vi "RFmx Update Sweep - TOI.vi"(8 "error in (no error)":errorcluster, 10 "Current Settings":T1={"Pin per Tone (dBm)"=0.0, "Equivalent Pin Power (dBm)"=0.0, "Frequency (Hz)"=0.0, "Tone Spacing (Hz)"=1000000.0}, 11 "RFmx Session in":refnum<k21>) -> (0 "error out":errorcluster, 3 "RFmx Session out":refnum<k21>)   [LabVIEW 2023]
uses:
  Controls/Data Cluster - Settings - TOI.ctl
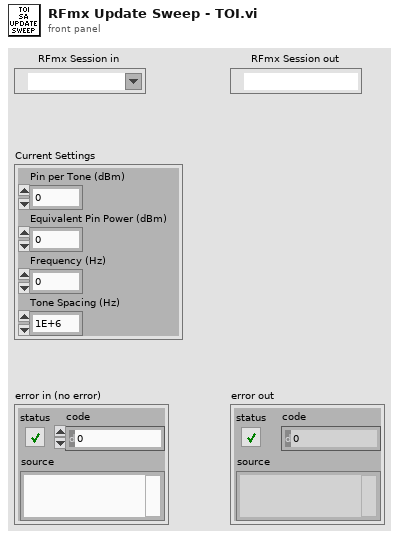
[diagram p1: front panel]
types:
  T1 = typedef "Data Cluster - Settings - TOI.ctl" = cluster{"Pin per Tone (dBm)":dbl, "Equivalent Pin Power (dBm)":dbl, "Frequency (Hz)":dbl, "Tone Spacing (Hz)":dbl}
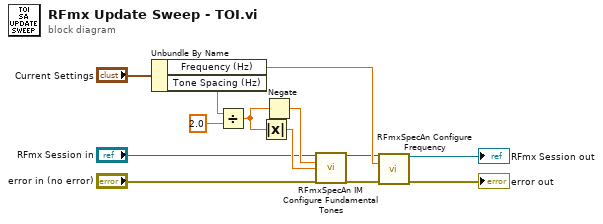
[diagram p0: block diagram]
diagram:
  n1 = Unbundle By Name("Current Settings") -> ("Frequency (Hz)"=w12:dbl, "Tone Spacing (Hz)"=w11:dbl)
  n2 = Divide(x=w11, y=2.0) -> (x/y=w7:dbl)
  n3 = Absolute Value(x=w7) -> (abs(x)=w6:dbl)
  n4 = Negate(x=w7) -> (-x=w8:dbl)
  n5 = call <vilib>:"RFmxSpecAn IM Configure Fundamental Tones.vi"("Instrument Handle In"="RFmx Session in", "Lower Tone Frequency (Hz)"=w8, "Upper Tone Frequency (Hz)"=w6) -> ("Instrument Handle Out"=w1:refnum<k21>)  [unwired: 11 in, 1 out]
  n6 = call <vilib>:"RFmxSpecAn Configure Frequency.vi"("Instrument Handle In"=w1, "Center Frequency (Hz)"=w12, "error in (no error)"="error in (no error)") -> ("Instrument Handle Out"=→"RFmx Session out":refnum<k21>, "error out"=→"error out":errorcluster)  [unwired: 11 in]
